vi "采配水启动器.vi"(8 "error in (no error)":errorcluster, 11 "启动/停止命令":T1(ring)) -> (0 "error out":errorcluster)   [LabVIEW 2016, in "质控单元V4.lvlib"]
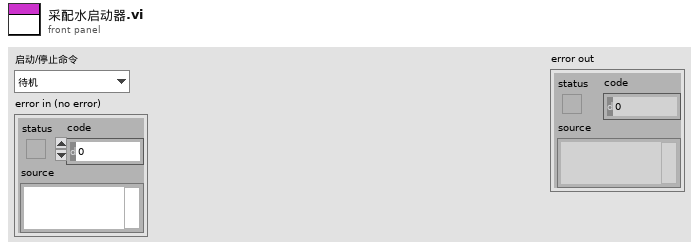
[diagram p1: front panel]
types:
  T1 = enum16{"待机", "水样测试（全流程）", "停止", "加标回收", "水样测试（简易流程）"}
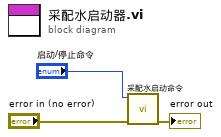
[diagram p0: block diagram]
diagram:
  n1 = call "采配水启动命令.vi"("error in (no error)"="error in (no error)", "启动/停止命令"="启动/停止命令") -> ("error out"=→"error out":errorcluster)  [unwired: 9 in]
